vi "Do.vi"(8 "error in (no error)":errorcluster, 10 "SetPower Message":refnum<class "SetPower Message.lvclass">, 11 "Actor.lvlib:Actor.lvclass":refnum<class "Execute.lvclass">) -> (0 "error out":errorcluster, 2 "SetPower Message":refnum<class "SetPower Message.lvclass">, 3 "Actor.lvlib:Actor.lvclass":refnum<class "Execute.lvclass">)   [LabVIEW 2018, in "QMH_Class.lvlib" / "TestManager.lvlib" / "SetPower Message.lvclass"]
uses:
  SetPower Message.lvclass
  Execute_class/Execute.lvclass
  SetPower Message.lvclass/SetPower Message.ctl
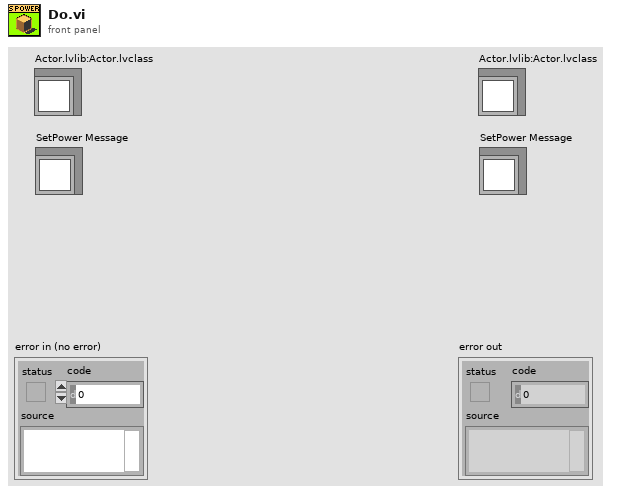
[diagram p1: front panel]
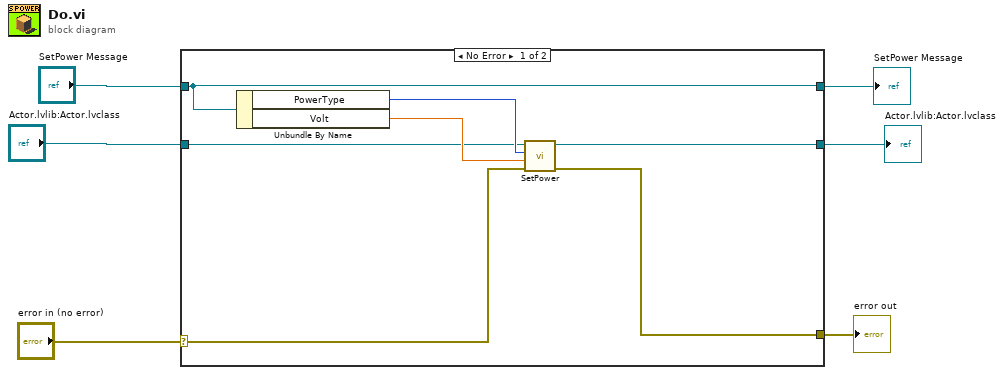
[diagram p0: block diagram]
diagram:
  n1 = case shown="No Error" "error in (no error)" {
    selector: "error in (no error)" -> [w7 w14]
    tunnel: "SetPower Message" -> [w8 w16]
    tunnel: [w11 w14] -> w5
    tunnel: [w10 w15] -> w4
    tunnel: "Actor.lvlib:Actor.lvclass" -> [w9 w15]
    tunnel: [w8 w16] -> w2
    frame No Error {
      n2 = Unbundle By Name(w8) -> ("PowerType"=w13:enum16{"Itech", "Keysight"}, "Volt"=w12:dbl)
      n3 = call-dynamic "SetPower.vi"("error in (no error)"=w7, "Numeric"=w12, "PowerType"=w13, "Execute"=w9) -> ("error out"=w11:errorcluster, "Execute"=w10:refnum<class "Execute.lvclass">)  [unwired: 6 in]
    }
    frame Error {
    }
  }
  "error out" <- w5
  "SetPower Message" <- w2
  "Actor.lvlib:Actor.lvclass" <- w4
